vi "删除界面.vi"(10 "删除前的界面":bool[][](array[boolean])) -> (0 "删除行数":dbl, 2 "删除后的界面":bool[][](array[boolean]))   [LabVIEW 2013]
panel:
  out "列数":i32
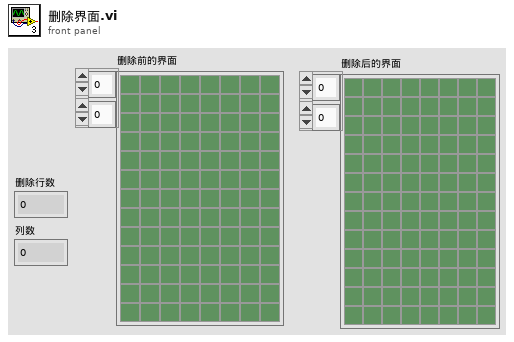
[diagram p1: front panel]
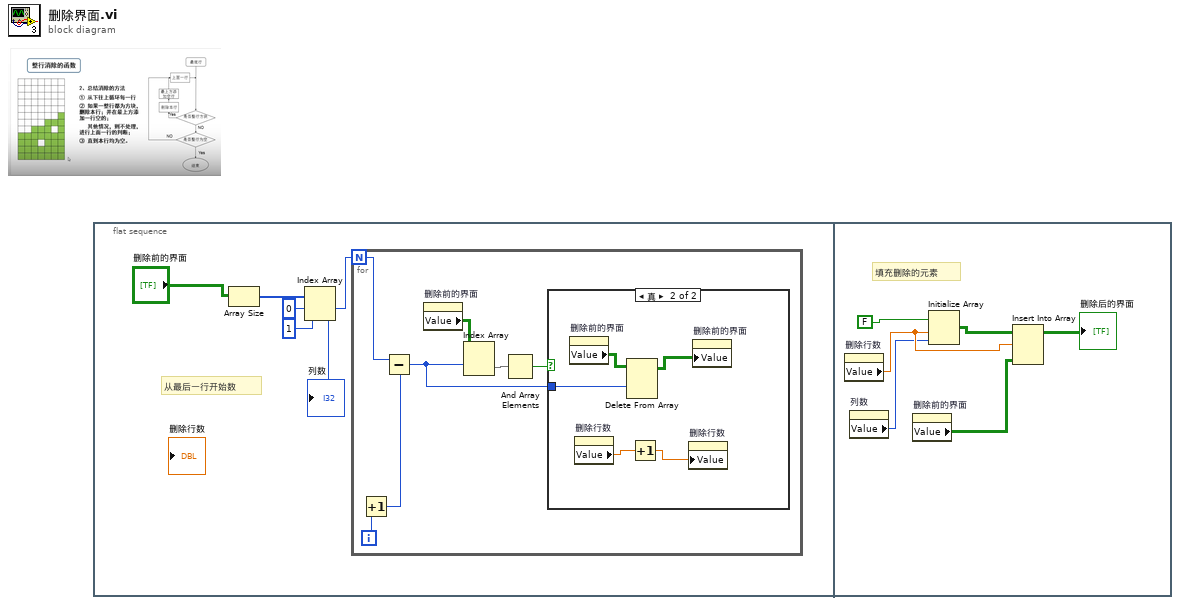
[diagram p0: block diagram]
diagram:
  n1 = flat-sequence {
    frame #0 {
      # "从最后一行开始数"
      n2 = Array Size(array="删除前的界面") -> (size(s)=w5:i32[])
      n3 = Index Array(array=w5, index #1=0 ("索引"), index #2=1 ("索引")) -> (element #1=w3:i32, element #2=→"列数":i32)
      n4 = for {
        N: w3 -> [w12]
        i -> [w13]
        n5 = Increment(x=w13) -> (x+1=w11:i32)
        n6 = Subtract(x=w12, y=w11) -> (x-y=w7:i32)
        n7 = property on="删除前的界面" class="Arr (严格)"() -> ("Value"=w10:bool[][])  [unwired: 2 in, 2 out]
        n8 = Index Array(array=w10, index (row)=w7) -> (element=w9:bool[])  [unwired: 1 in]
        n9 = And Array Elements(Boolean array=w9) -> (logical AND=w8:bool)
        n10 = case shown="真" w8 {
          tunnel: w7 -> [_ w17]
          frame False {
          }
          frame True {
            n11 = property on="删除前的界面" class="Arr (严格)"() -> ("Value"=w18:bool[][])  [unwired: 2 in, 2 out]
            n12 = property on="删除行数" class="DigNum (严格)"() -> ("Value"=w15:dbl)  [unwired: 2 in, 2 out]
            n13 = Delete From Array(array=w18, index (row)=w17) -> (array with subset deleted=w16:bool[][])  [unwired: 2 in, 1 out]
            n14 = Increment(x=w15) -> (x+1=w14:dbl)
            n15 = property on="删除行数" class="DigNum (严格)"("Value"=w14) -> ()  [unwired: 2 in, 2 out]
            n16 = property on="删除前的界面" class="Arr (严格)"("Value"=w16) -> ()  [unwired: 2 in, 2 out]
          }
        }
      }
    }
    frame #1 {
      # "填充删除的元素"
      n17 = property on="删除行数" class="DigNum (严格)"() -> ("Value"=w22:dbl)  [unwired: 2 in, 2 out]
      n18 = property on="列数" class="DigNum (严格)"() -> ("Value"=w19:i32)  [unwired: 2 in, 2 out]
      n19 = property on="删除前的界面" class="Arr (严格)"() -> ("Value"=w21:bool[][])  [unwired: 2 in, 2 out]
      n20 = Initialize Array(FALSE, w22, w19) -> (w23:bool[][])
      n21 = Insert Into Array(array=w23, index (row)=w22, new element=w21) -> (→"删除后的界面":bool[][])  [unwired: 1 in]
    }
  }
